vi "Pause.vi"(8 "error in (no error)":errorcluster, 11 "State in":T1={"State"=enum."Idle", "Start Time"=timestamp(0 s since 1904-01-01), "Configuration"={"Cycle Period"=0.0, "PID 2 Parameters"={"Input Device"=enum."4-20mA", "Output Device"=enum."Default", "Setpoint"=0.0, "PID gains"={"proportional gain (Kc)"=0.0, "integral time (Ti, min)"=0.0, "derivative time (Td, min)"=100.0}, "output range"={"output low"=0.0, "output high"=1.0}}, "Manual Entry"=0.0, "Auto?"=TRUE, "4-20mA Input Settings"={"Input Channel "=0}, "4-20mA Out Settings"={"Output DAQ Task"=""}, "Input Channel Tag Name "=""}, "Current Time"=timestamp(0 s since 1904-01-01), "PID 1 Parameters"={"Setpoint"=0.0, "PID gains"={"proportional gain (Kc)"=1.0, "integral time (Ti, min)"=0.01, "derivative time (Td, min)"=0.0}}, "First Iteration"=TRUE, "Data"={"4-20mA Input"=0.0, "PID 2 Process Variable"=0.0, "PID 2 Output"=0.0, "4-20mA Output"=0.0}, "Process Name"="", "Pump On?"=enum."Off", "Input Error"=FALSE, "Output Error"=FALSE, "Log Started"=FALSE, "Current Setpoint"=0.0} {"Configuration"."PID 2 Parameters"."output range"."output low" format="%.2f"; "Configuration"."PID 2 Parameters"."output range"."output high" min=0.0 max=100.0 format="%.2f"; "Configuration"."PID 2 Parameters"."PID gains"."derivative time (Td, min)" format="%.3f"; "Configuration"."PID 2 Parameters"."PID gains"."integral time (Ti, min)" format="%.3f"; "Configuration"."PID 2 Parameters"."PID gains"."proportional gain (Kc)" format="%.3f"; "PID 1 Parameters"."PID gains"."derivative time (Td, min)" format="%.3f"; "PID 1 Parameters"."PID gains"."integral time (Ti, min)" format="%.3f"; "PID 1 Parameters"."PID gains"."proportional gain (Kc)" format="%.3f"}) -> (0 "error out":errorcluster, 3 "State out":T1={"State"=enum."Idle", "Start Time"=timestamp(0 s since 1904-01-01), "Configuration"={"Cycle Period"=0.0, "PID 2 Parameters"={"Input Device"=enum."4-20mA", "Output Device"=enum."Default", "Setpoint"=0.0, "PID gains"={"proportional gain (Kc)"=0.0, "integral time (Ti, min)"=0.0, "derivative time (Td, min)"=100.0}, "output range"={"output low"=0.0, "output high"=1.0}}, "Manual Entry"=0.0, "Auto?"=TRUE, "4-20mA Input Settings"={"Input Channel "=0}, "4-20mA Out Settings"={"Output DAQ Task"=""}, "Input Channel Tag Name "=""}, "Current Time"=timestamp(0 s since 1904-01-01), "PID 1 Parameters"={"Setpoint"=0.0, "PID gains"={"proportional gain (Kc)"=1.0, "integral time (Ti, min)"=0.01, "derivative time (Td, min)"=0.0}}, "First Iteration"=FALSE, "Data"={"4-20mA Input"=0.0, "PID 2 Process Variable"=0.0, "PID 2 Output"=0.0, "4-20mA Output"=0.0}, "Process Name"="", "Pump On?"=enum."Off", "Input Error"=FALSE, "Output Error"=FALSE, "Log Started"=FALSE, "Current Setpoint"=0.0} {"Configuration"."PID 2 Parameters"."output range"."output low" format="%.2f"; "Configuration"."PID 2 Parameters"."output range"."output high" min=0.0 max=100.0 format="%.2f"; "Configuration"."PID 2 Parameters"."PID gains"."derivative time (Td, min)" format="%.3f"; "Configuration"."PID 2 Parameters"."PID gains"."integral time (Ti, min)" format="%.3f"; "Configuration"."PID 2 Parameters"."PID gains"."proportional gain (Kc)" format="%.3f"; "PID 1 Parameters"."PID gains"."derivative time (Td, min)" format="%.3f"; "PID 1 Parameters"."PID gains"."integral time (Ti, min)" format="%.3f"; "PID 1 Parameters"."PID gains"."proportional gain (Kc)" format="%.3f"})   [LabVIEW 2021, in "4-20mA Module.lvlib" / "4-20mA Module Engine.lvlib"]
uses:
  4-20mA Module Engine.lvlib
  State Cluster.ctl
  State Enum.ctl
  Pressure Transmitter/Pressure Transmitter Device Settings.ctl
  Pressure Reg Module/Pressure Regulator Device Settings.ctl
  Measure Instrument/PID 1 Parameters Cluster.ctl
  Pressure Reg Module/Pressure Regulator Library.lvlib
  Pressure Transmitter/Pressure Transmitter Library.lvlib
panel:
  # "Instrument Settings"
  # "Instrument Settings"
  # "Instrument Settings"
  # "Instrument Settings"
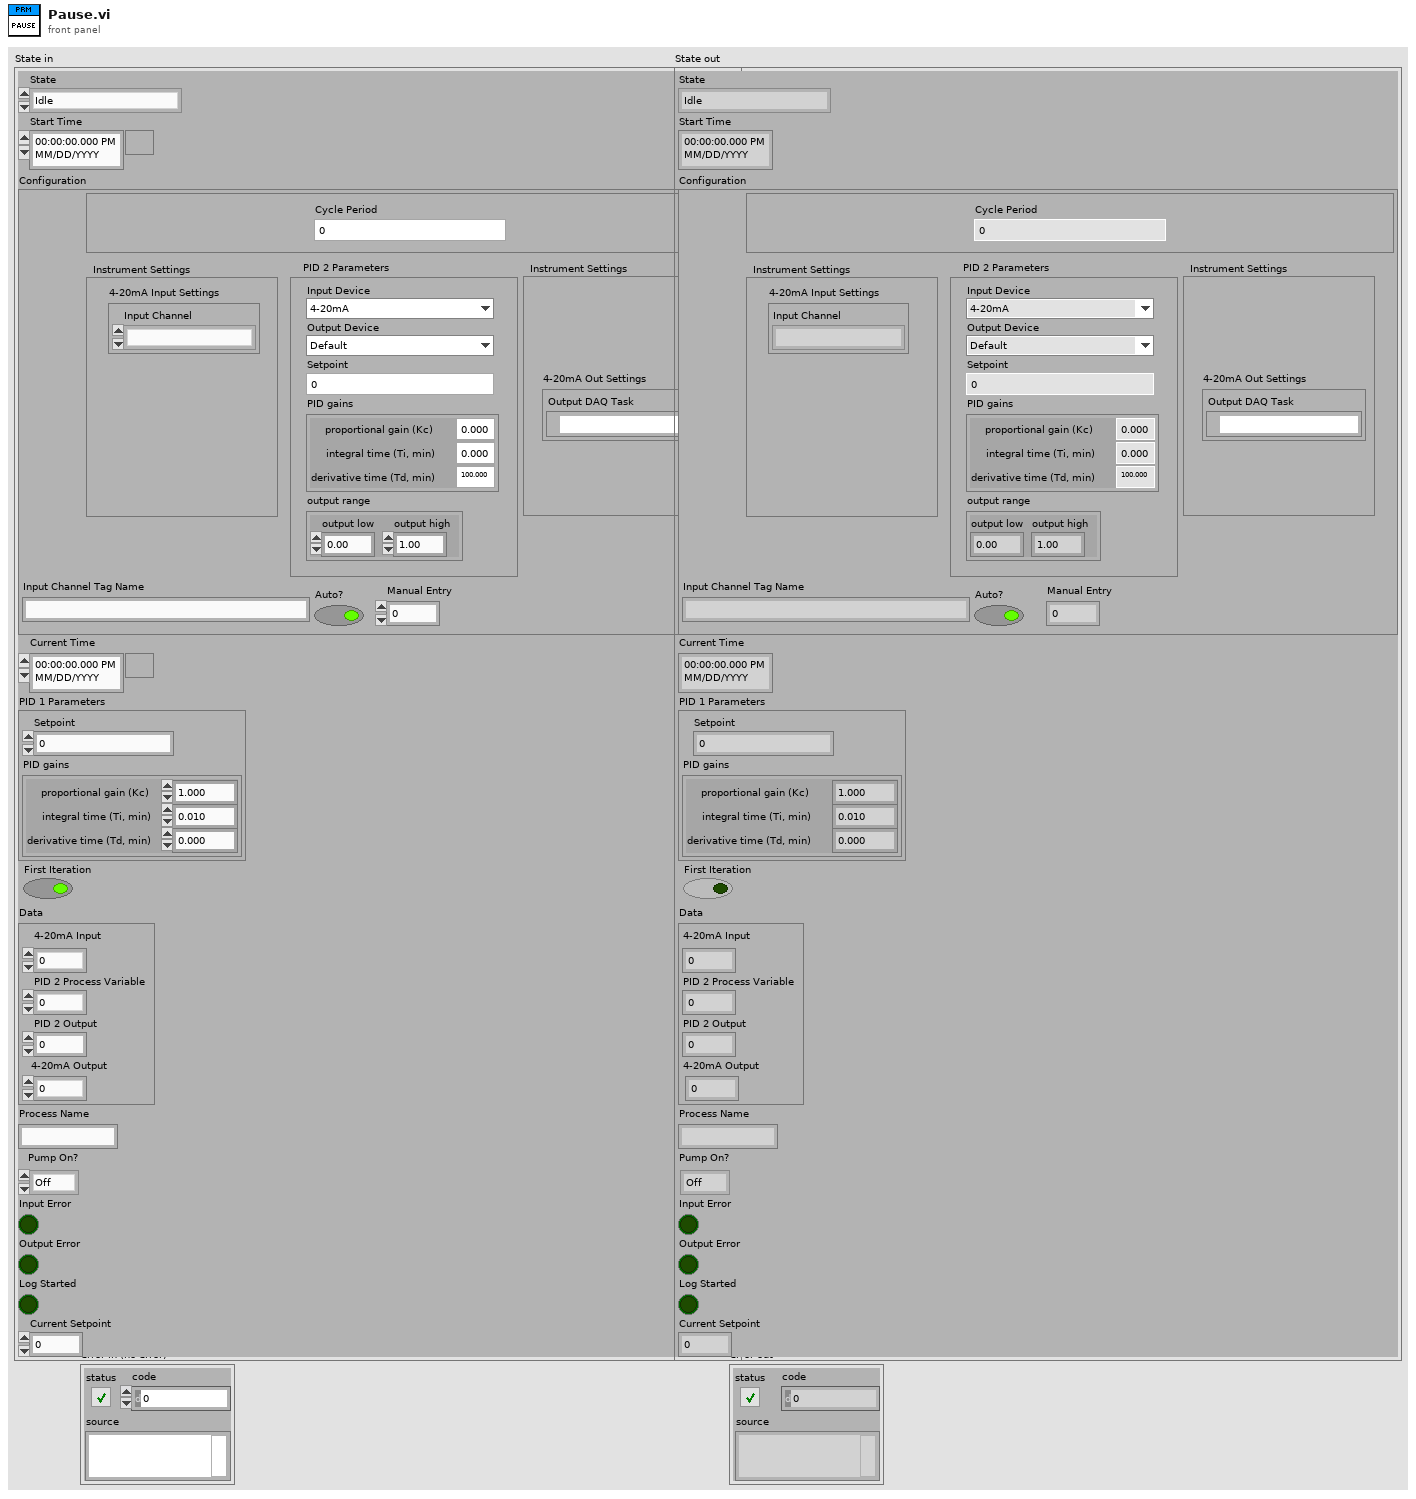
[diagram p1: front panel]
types:
  T1 = typedef "4-20mA Module.lvlib/4-20mA Module Engine.lvlib/State Cluster.ctl" = cluster{"State":T2, "Start Time":timestamp, "Configuration":cluster{"Cycle Period":dbl, "PID 2 Parameters":cluster{"Input Device":enum16{"Default", "4-20mA"}, "Output Device":enum16{"Default", "Equilibar Pressure Reg", "Flow Regulator"}, "Setpoint":dbl, "PID gains":cluster{"proportional gain (Kc)":dbl, "integral time (Ti, min)":dbl, "derivative time (Td, min)":dbl}, "output range":cluster{"output low":dbl, "output high":dbl}}, "Manual Entry":dbl, "Auto?":bool, "4-20mA Input Settings":T3, "4-20mA Out Settings":T4, "Input Channel Tag Name ":string}, "Current Time":timestamp, "PID 1 Parameters":T5, "First Iteration":bool, "Data":cluster{"4-20mA Input":dbl, "PID 2 Process Variable":dbl, "PID 2 Output":dbl, "4-20mA Output":dbl}, "Process Name":string, "Pump On?":enum16{"Off", "On", "Not Initialized"}, "Input Error":bool, "Output Error":bool, "Log Started":bool, "Current Setpoint":dbl}
  T2 = typedef "4-20mA Module.lvlib/4-20mA Module Engine.lvlib/State Enum.ctl" = enum16{"Measuring", "Idle", "Paused"}
  T3 = typedef "Pressure Transmitter Library.lvlib/Pressure Transmitter Device Settings.ctl" = cluster{"Input Channel ":u16}
  T4 = typedef "Pressure Regulator Library.lvlib/Pressure Regulator Device Settings.ctl" = cluster{"Output DAQ Task":refnum<k21>}
  T5 = typedef "PID 1 Parameters Cluster.ctl" = cluster{"Setpoint":dbl, "PID gains":cluster{"proportional gain (Kc)":dbl, "integral time (Ti, min)":dbl, "derivative time (Td, min)":dbl}}
  T6 = enum16{"Default", "Equilibar Pressure Reg", "Flow Regulator"}
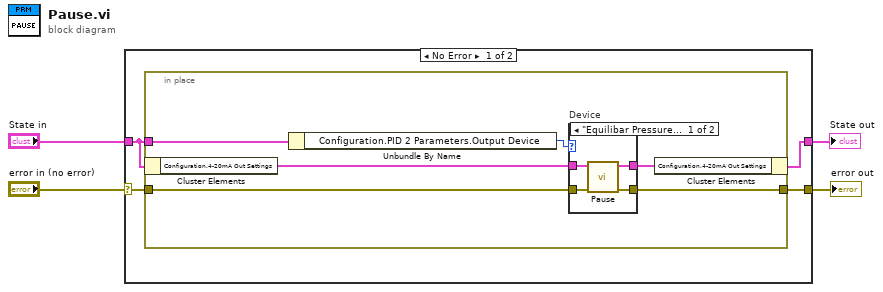
[diagram p0: block diagram]
diagram:
  n1 = case shown="No Error" "error in (no error)" {
    selector: "error in (no error)" -> [w7 w22]
    tunnel: [w8 w22] -> w3
    tunnel: "State in" -> [w6 w21]
    tunnel: [w5 w21] -> w1
    frame No Error {
      n2 = in-place {
        in-place-border: w6 -> [w14]
        in-place-border: [w13] -> w8
        in-place-border: w7 -> [w12]
        n3 = in-place-cluster #1(w6) -> ("Configuration.4-20mA Out Settings"=w10:T4)
        n4 = Unbundle By Name(w14) -> ("Configuration.PID 2 Parameters.Output Device"=w11:T6)
        n5 = case "Device" shown="\"Equilibar Pressure Reg\"" w11 {
          tunnel: [w17 w20] -> w13
          tunnel: [w18 w19] -> w9
          tunnel: w12 -> [w16 w20]
          tunnel: w10 -> [w15 w19]
          frame "Equilibar Pressure Reg" {
            n6 = call "Pause.vi"("error in"=w16, "4-20mA Out Settings In"=w15) -> ("error out"=w17:errorcluster, "4-20mA Out Settings Out"=w18:T4)  [unwired: 8 in]
          }
          frame "Default", Default {
          }
        }
        n7 = in-place-cluster #1("Configuration.4-20mA Out Settings"=w9) -> (w5:T1)
      }
    }
    frame Error {
    }
  }
  "error out" <- w3
  "State out" <- w1
